vi "2. MotorTest.vi"(1 "Stop Button":bool, 8 "error in (no error)":errorcluster, 10 "Speed (PWM)":dbl(slide) scale=-100.0..100.0) -> (0 "error out":errorcluster, 2 "MotorEncoder (deg)":dbl)   [LabVIEW 2019, in "SJCube.lvlib"]
uses:
  SJCube.lvlib
panel:
  in  "Reset Counter":bool
  out "gearedMotorEncoder (deg)":dbl
  # "ATTENTION:\n\nDO THIS EXP. ONLY WHEN THE PENDULUM \nIS \"NOT\" INSTALLED"
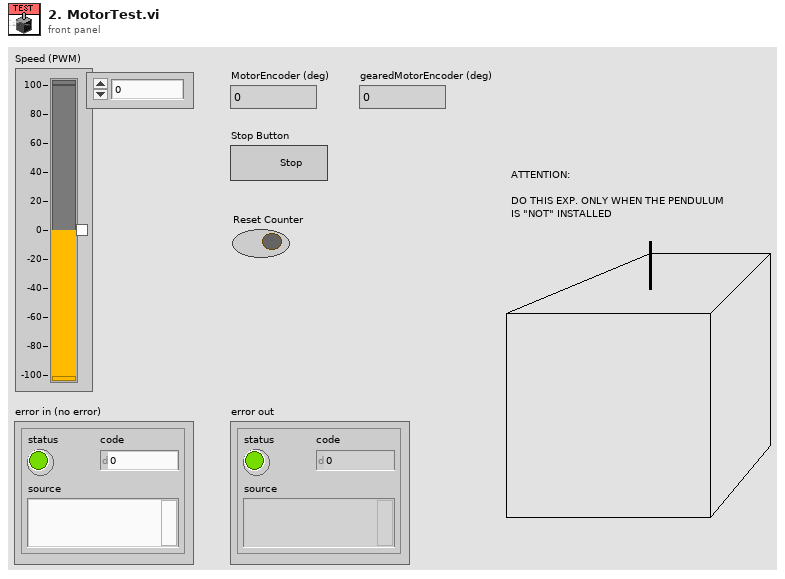
[diagram p1: front panel]
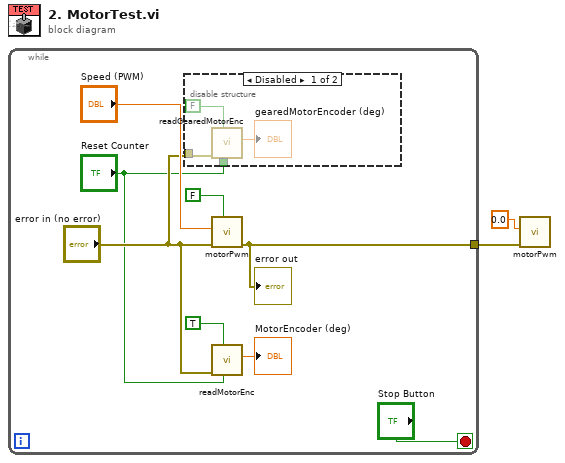
[diagram p0: block diagram]
diagram:
  n1 = while {
    tunnel: [w6] -> w2
    stop <- "Stop Button" stop-if-true
    n2 = disable-structure shown="Disabled" {
      disable-tunnel: "error in (no error)" -> [w14 _]
      disable-tunnel: "Reset Counter" -> [w11 _]
      frame Disabled {
        n3 = call "readGearedMotorEnc.vi"("Reset Counter"=w11, "Reverse ENC?"=FALSE, "error in (no error)"=w14) -> ("gearedMotorEncoder (deg)"=→"gearedMotorEncoder (deg)":dbl)  [unwired: 7 in, 1 out]
      }
      frame Enabled {
      }
    }
    n4 = call "motorPwm.vi"("reverse?"=FALSE, "error in (no error)"="error in (no error)", "Speed (PWM)"="Speed (PWM)") -> ("error out"=w6:errorcluster)  [unwired: 8 in]
    "error out" <- w6
    n5 = call "readMotorEnc.vi"("Reset Counter"="Reset Counter", "Reverse ENC?"=TRUE, "error in (no error)"="error in (no error)") -> ("MotorEncoder (deg)"=→"MotorEncoder (deg)":dbl)  [unwired: 7 in, 1 out]
  }
  n6 = call "motorPwm.vi"("error in (no error)"=w2, "Speed (PWM)"=0.0) -> ()  [unwired: 9 in, 1 out]
